vi "DFD Plot Step Response.vi"(5 "output option":u16(ring) items=["Auto", "Floating-Point Only", "Fixed-Point Only"], 6 "fs [Hz]":dbl=-1.0 format="%.2f", 7 "# points":i32=-1, 8 "error in (no error)":errorcluster, 11 "filter in":T1={"mSRate_Fs"=1.0, "mSRate_Version"="2.0", "mSRate_Comments"="", "mSRate_OrgCoef"={"type"=enum."Undefined", "gain"=1.0, "coef a (k)"=[], "coef b (v)"=[]}, "mSRate_CurCoef"={"type"=enum."Undefined", "gain"=1.0, "coef a (k)"=[], "coef b (v)"=[]}, "mSRate_Quantized?"=FALSE, "mSRate_QCoef"={"type"=enum."Undefined", "gain"=1.0, "coef a (k)"=[], "coef b (v)"=[]}, "mSRate_QSettings"=[], "mSRate_Order"=0, "mSRate_Scaling"={"mSRate_ScaleByPowerOf2?"=FALSE, "mSRate_ScaleType"=enum."No Norm"}} {"mSRate_QSettings"."source" items=["Coef a/k"=0, "Coef b/v"=7, "Input"=1, "Output"=2, "Multiplicand"=3, "Product"=4, "Sum"=5, "Delay"=6, "Gain"=8]}) -> (0 "error out":errorcluster, 2 "step response":T7(graph), 3 "filter out":T1={"mSRate_Fs"=1.0, "mSRate_Version"="2.0", "mSRate_Comments"="", "mSRate_OrgCoef"={"type"=enum."Undefined", "gain"=1.0, "coef a (k)"=[], "coef b (v)"=[]}, "mSRate_CurCoef"={"type"=enum."Undefined", "gain"=1.0, "coef a (k)"=[], "coef b (v)"=[]}, "mSRate_Quantized?"=FALSE, "mSRate_QCoef"={"type"=enum."Undefined", "gain"=1.0, "coef a (k)"=[], "coef b (v)"=[]}, "mSRate_QSettings"=[], "mSRate_Order"=0, "mSRate_Scaling"={"mSRate_ScaleByPowerOf2?"=FALSE, "mSRate_ScaleType"=enum."No Norm"}} {"mSRate_QSettings"."source" items=["Coef a/k"=0, "Coef b/v"=7, "Input"=1, "Output"=2, "Multiplicand"=3, "Product"=4, "Sum"=5, "Delay"=6, "Gain"=8]})   [LabVIEW 2017, in "NI_DigFilterLicensed.lvlib"]
doc: "Plots the step response of a filter."
uses:
  <vilib>/addons/Digital Filter Design/NI_DigFilterLicensed.lvlib
  <vilib>/addons/Digital Filter Design/_Objects.llb/DFD Filter Obj.ctl
  <vilib>/addons/Digital Filter Design/_Objects.llb/DFD Filter Coef.ctl
  <vilib>/addons/Digital Filter Design/_Objects.llb/DFD Filter Structure Type Selector.ctl
  <vilib>/addons/Digital Filter Design/_Objects.llb/dfd_Internal Quantization Settings.ctl
  <vilib>/addons/Digital Filter Design/_Objects.llb/dfd_Internal Quantization Srcs.ctl
  <vilib>/addons/Digital Filter Design/_Objects.llb/DFD Coef Norm Type.ctl
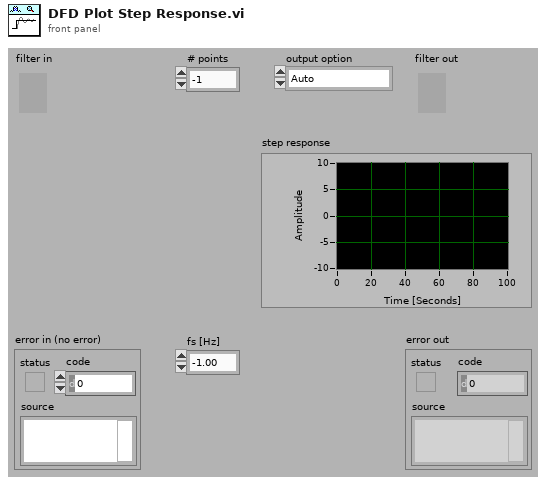
[diagram p1: front panel]
types:
  T1 = typedef "NI_DigFilterLicensed.lvlib/DFD Filter Obj.ctl" = cluster{"mSRate_Fs":dbl, "mSRate_Version":string, "mSRate_Comments":string, "mSRate_OrgCoef":T2, "mSRate_CurCoef":T2, "mSRate_Quantized?":bool, "mSRate_QCoef":T2, "mSRate_QSettings":T4[], "mSRate_Order":i32, "mSRate_Scaling":cluster{"mSRate_ScaleByPowerOf2?":bool, "mSRate_ScaleType":T6}}
  T2 = typedef "NI_DigFilterLicensed.lvlib/DFD Filter Coef.ctl" = cluster{"type":T3, "gain":dbl, "coef a (k)":dbl[], "coef b (v)":dbl[]}
  T3 = typedef "NI_DigFilterLicensed.lvlib/DFD Filter Structure Type Selector.ctl" = enum16{"Undefined", "FIR Direct Form", "FIR Direct Form Transposed", "FIR Symmetric", "FIR Antisymmetric", "IIR Direct Form I", "IIR Direct Form I Transposed", "IIR Direct Form II", "IIR Direct Form II Transposed", "IIR Cascaded Second Order Sections Form I", "IIR Cascaded Second Order Sections Form I Transposed", "IIR Cascaded Second Order Sections Form II", "IIR Cascaded Second Order Sections Form II Transposed", "Lattice Allpass (basic sections)", "Lattice Allpass (one multiplier sections)", "Lattice Allpass (normalized sections)", "Lattice AR (basic sections)", "Lattice AR (one multiplier sections)", "Lattice AR (normalized sections)", "Lattice MA (minimum phase)", "Lattice MA (maximum phase)", "Lattice ARMA (basic sections)", "Lattice ARMA (one multiplier sections)", "Lattice ARMA (normalized sections)"}
  T4 = typedef "NI_DigFilterLicensed.lvlib/dfd_Internal Quantization Settings.ctl" = cluster{"source":T5, "wl":i16, "iwl":i16, "overflow mode":enum16{"Saturation", "Wrap"}, "rounding mode":enum16{"Nearest", "Truncation"}, "signed?":bool}
  T5 = typedef "NI_DigFilterLicensed.lvlib/dfd_Internal Quantization Srcs.ctl" = u16
  T6 = typedef "NI_DigFilterLicensed.lvlib/DFD Coef Norm Type.ctl" = enum16{"No Norm", "Time Domain 1-Norm", "Time Domain 2-Norm", "Time Domain Inf-Norm"}
  T7 = cluster{"t0":dbl, "dt":dbl, "amplitudes":dbl[]}[]
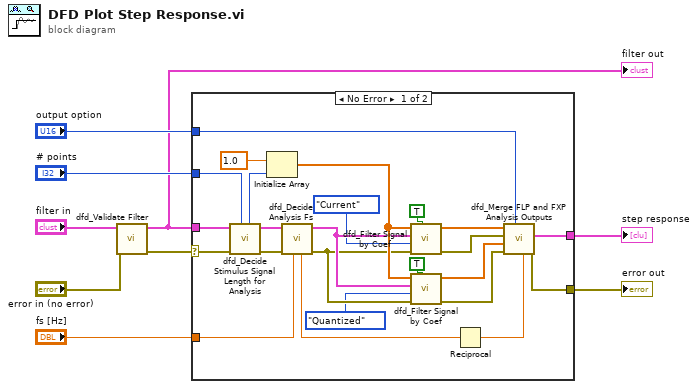
[diagram p0: block diagram]
diagram:
  n1 = call <vilib>:"dfd_Validate Filter.vi"("error in (no error)"="error in (no error)", "filter in"="filter in") -> ("error out"=w2:errorcluster, "filter out"=w1:T1)  [unwired: 1 in, 7 out]
  "filter out" <- w1
  n2 = case shown="No Error" w2 {
    selector: w2 -> [w18 w34]
    tunnel: w1 -> [w22 _]
    tunnel: "# points" -> [w20 _]
    tunnel: [w29 w34] -> w8
    tunnel: [w16 _] -> w7
    tunnel: "fs [Hz]" -> [w33 _]
    tunnel: "output option" -> [w30 _]
    frame No Error {
      n3 = call <vilib>:"dfd_Decide Stimulus Signal Length for Analysis.vi"("#points in"=w20, "error in (no error)"=w18, "filter in"=w22) -> ("error out"=w17:errorcluster, "filter out"=w21:T1, "#points out"=w19:i32)  [unwired: 6 out]
      n4 = Initialize Array(1.0 ("amplitude"), w19) -> (w31:dbl[])
      n5 = call <vilib>:"dfd_Decide Analysis Fs.vi"("fs in [Hz]"=w33, "error in (no error)"=w17, "filter in"=w21) -> ("error out"=w14:errorcluster, "filter out"=w15:T1, "fs out [Hz]"=w32:dbl)  [unwired: 6 out]
      n6 = call <vilib>:"dfd_Filter Signal by Coef.vi"("initH?"=TRUE, "error in(no error)"=w14, "coef source"=enum16{"Original", "Current", "Quantized"}."Current", "filter"=w15, "x"=w31) -> ("error out"=w25:errorcluster, "filtered x"=w26:dbl[])  [unwired: 1 in, 4 out]
      n7 = call <vilib>:"dfd_Filter Signal by Coef.vi"("initH?"=TRUE, "error in(no error)"=w14, "coef source"=enum16{"Original", "Current", "Quantized"}."Quantized", "filter"=w15, "x"=w31) -> ("error out"=w28:errorcluster, "filtered x"=w24:dbl[])  [unwired: 1 in, 4 out]
      n8 = Reciprocal(x=w32) -> (1/x=w23:dbl)
      n9 = call <vilib>:"dfd_Merge FLP and FXP Analysis Outputs.vi"("delta"=w23, "output option"=w30, "error in FXP"=w28, "response FXP"=w24, "error in FLP"=w25, "response FLP"=w26) -> ("error out"=w29:errorcluster, "time responses"=w16:T7)  [unwired: 4 out]
    }
    frame Error {
    }
  }
  "error out" <- w8
  "step response" <- w7
